vi "LvIRKit_RegistButton_Panel.vi"(11 "IRKit IP":string) -> (1 "irdata":T1, 2 "Cancel?":bool)   [LabVIEW 2014]
uses:
  LvIRKit_rsc_IRData_typedef.ctl
panel:
  in  "Btn Scan":bool
  in  "Btn Cancel":bool
  # "IRKit に向けてリモコンボタンを軽く押してください。\nLEDが点滅したら読み取りボタンを押してください。"
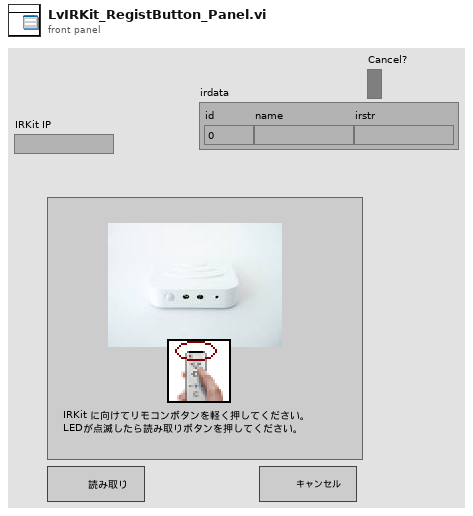
[diagram p1: front panel]
types:
  T1 = typedef "LvIRKit_rsc_IRData_typedef.ctl" = cluster{"id":i32, "name":string, "irstr":string}
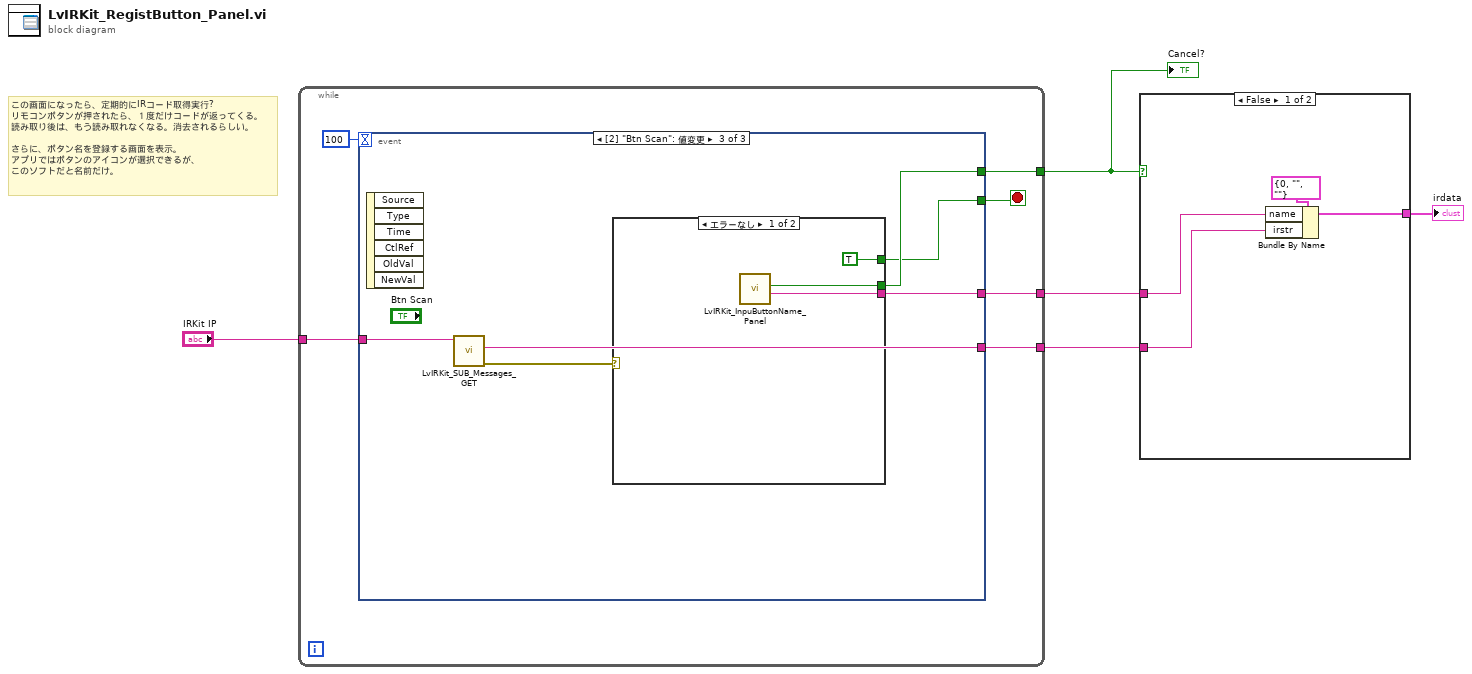
[diagram p0: block diagram]
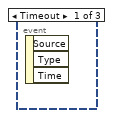
[diagram p2: hidden frame]
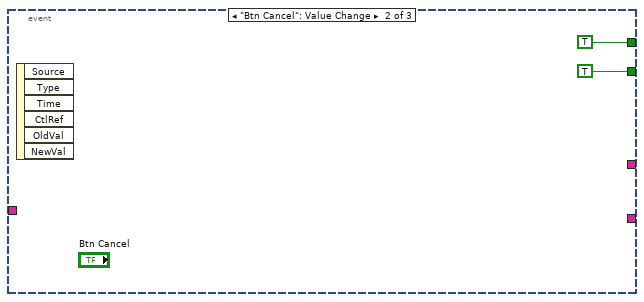
[diagram p3: hidden frame]
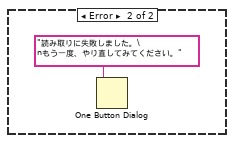
[diagram p4: hidden frame]
diagram:
  # "この画面になったら、定期的にIRコード取得実行?\nリモコンボタンが押されたら、１度だけコードが返ってくる。\n読み取り後は、もう読み取れなくなる。消去されるらしい。\n\nさらに、ボタン名を登録する画面を表示。\nアプリではボタンのアイコンが選択できるが、\nこのソフトだと名前だけ。"
  n1 = while {
    tunnel: [w9] -> w4
    tunnel: "IRKit IP" -> [w8]
    tunnel: [w7] -> w2
    tunnel: [w6] -> w1
    stop <- w10 stop-if-true
    n2 = event shown="[2] \"Btn Scan\": 値変更" {
      selector: _ -> [_ _ _]
      dyn-events: _ -> [_ _ _]
      timeout: 100 -> [_ _ _]
      tunnel: [_ TRUE w14] -> w10
      tunnel: [_ TRUE w15] -> w9
      tunnel: w8 -> [_ _ w19]
      tunnel: [_ _ w17] -> w7
      tunnel: [_ _ w16] -> w6
      event Timeout {
        n3 = event-data() -> ()  [unwired: 1 in, 3 out]
      }
      event "Btn Cancel": Value Change {
        n4 = event-data() -> ()  [unwired: 1 in, 6 out]
      }
      event "Btn Scan": Value Change {
        n5 = event-data() -> ()  [unwired: 1 in, 6 out]
        n6 = call "LvIRKit_SUB_Messages_GET.vi"("IRKit IP address"=w19) -> ("error out"=w18:errorcluster, "Message"=w17:string)  [unwired: 9 in]
        n7 = case shown="エラーなし" w18 {
          tunnel: [w22 _] -> w15
          tunnel: [w21 _] -> w16
          tunnel: [TRUE _] -> w14
          frame No Error {
            n8 = call "LvIRKit_InpuButtonName_Panel.vi"() -> ("buttunName"=w21:string, "Cancel?"=w22:bool)  [unwired: 10 in]
          }
          frame Error {
            n9 = One Button Dialog(message="読み取りに失敗しました。\nもう一度、やり直してみてください。" ("メッセージ")) -> ()  [unwired: 1 in, 1 out]
          }
        }
      }
    }
  }
  "Cancel?" <- w4
  n10 = case shown="FALSE" w4 {
    tunnel: [w26 _] -> w5
    tunnel: w2 -> [w24 _]
    tunnel: w1 -> [w25 _]
    frame False {
      n11 = Bundle By Name(cluster=T1 {"id"=0, "name"="", "irstr"=""} ("irdata"), "name"=w25, "irstr"=w24) -> (w26:T1)
    }
    frame True {
      # "Cancel"
    }
  }
  "irdata" <- w5
